vi "Flatten Cluster To CfgTable(with DataName).vi"(8 "error in (no error)":errorcluster, 10 "ParentName":string, 11 "Cluster Configuration Typedef":variant) -> (0 "error out":errorcluster, 2 "CfgTable Row Header":string[](array[string]), 3 "CfgTable Row":string[](array[string]))   [LabVIEW 2017, in "ClusterCfgTable.lvlib"]
uses:
  ClusterCfgTable.lvlib
panel:
  in  "ConfigStrings Typedef":string[](array[string])
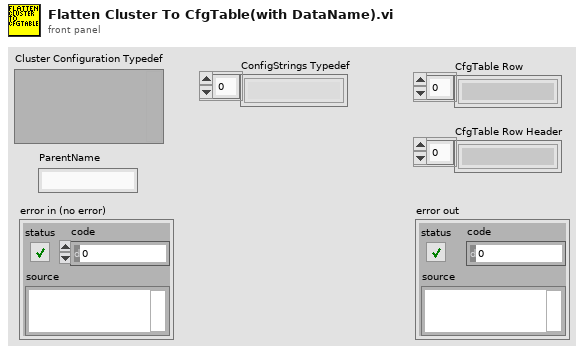
[diagram p1: front panel]
types:
  T1 = typedef "Type Descriptor Enumeration__ogtk.ctl" = enum8{"<Null>", "I8", "I16", "I32", "I64", "U8", "U16", "U32", "U64", "SGL", "DBL", "EXT", "CSG", "CDB", "CXT", "0x0F", "0x10", "0x11", "0x12", "0x13", "0x14", "Enum U8", "Enum U16", "Enum U32", "Enum U64", "SGL PQ", "DBL PQ", "EXT PQ", "CSG PQ", "CDB PQ", "CXT PQ", "0x1F", "0x20", "Boolean", "0x22", "0x23", "0x24", "0x25", "0x26", "0x27", "0x28", "0x29", "0x2A", "0x2B", "0x2C", "0x2D", "0x2E", "0x2F", "String", "0x31", "Path", "Pict", "0x34", "0x35", "0x36", "DAQ", "0x38", "0x39", "0x3A", "0x3B", "0x3C", "0x3D", "0x3E", "0x3F", "Array", "0x41", "0x42", "0x43", "0x44", "0x45", "0x46", "0x47", "0x48", "0x49", "0x4A", "0x4B", "0x4C", "0x4D", "0x4E", "0x4F", "Cluster", "0x51", "0x52", "Variant", "Waveform", "0x55", "0x56", "0x57", "0x58", "0x59", "0x5A", "0x5B", "0x5C", "0x5D", "0x5E", "0x5F", "0x60", "0x61", "0x62", "0x63", "0x64", "0x65", "0x66", "0x67", "0x68", "0x69", "0x6A", "0x6B", "0x6C", "0x6D", "0x6E", "0x6F", "Refnum"}
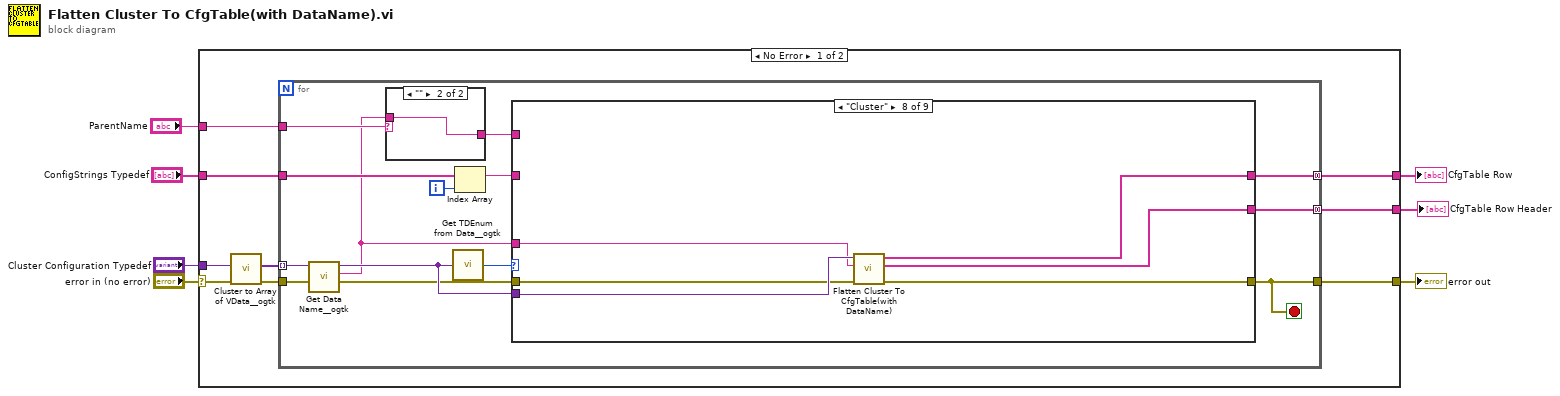
[diagram p0: block diagram]
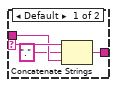
[diagram p2: hidden frame]
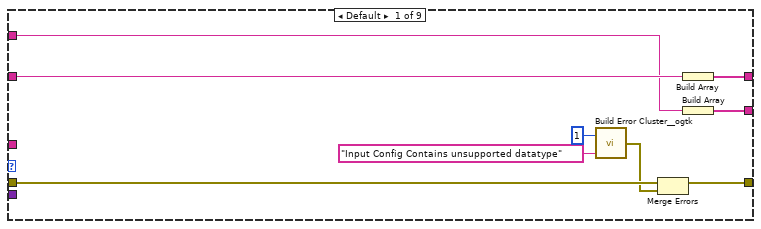
[diagram p3: hidden frame]
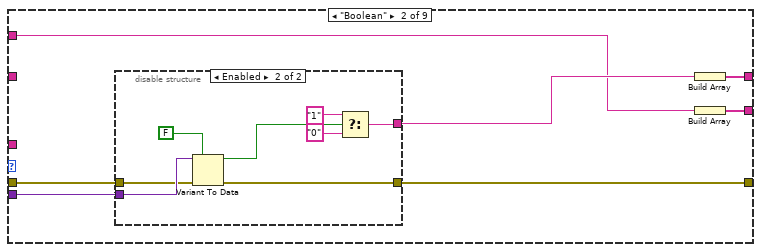
[diagram p4: hidden frame]
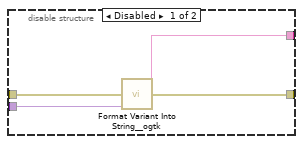
[diagram p5: hidden frame]
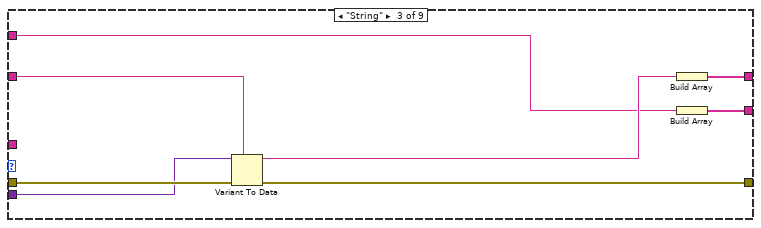
[diagram p6: hidden frame]
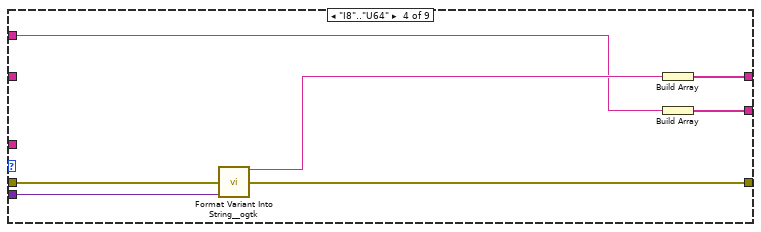
[diagram p7: hidden frame]
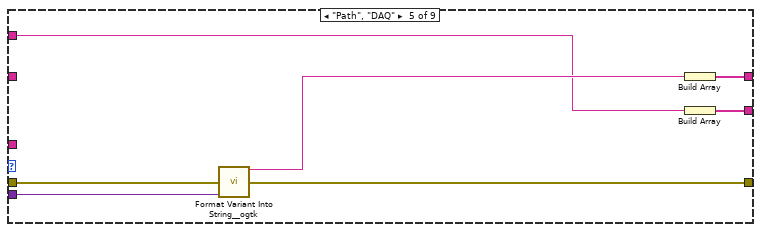
[diagram p8: hidden frame]
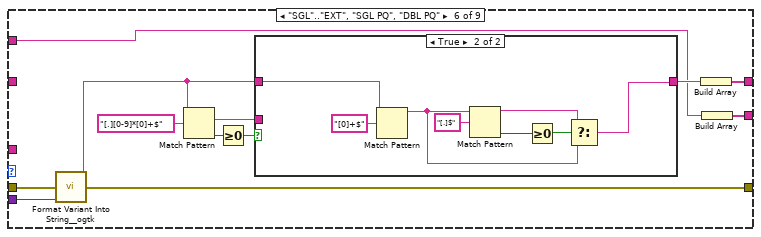
[diagram p9: hidden frame]
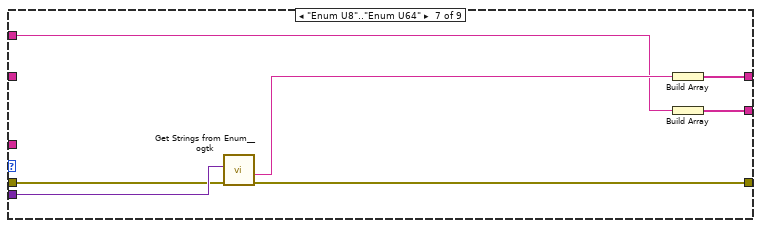
[diagram p11: hidden frame]
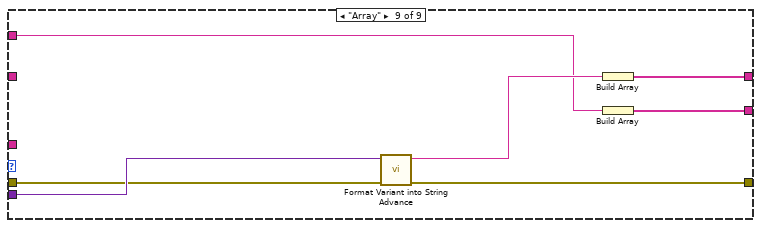
[diagram p12: hidden frame]
diagram:
  n1 = case shown="No Error" "error in (no error)" {
    selector: "error in (no error)" -> [w14 w128]
    tunnel: [w16 w128] -> w7
    tunnel: "Cluster Configuration Typedef" -> [w12 _]
    tunnel: [w11 w127] -> w4
    tunnel: "ConfigStrings Typedef" -> [w10 w127]
    tunnel: "ParentName" -> [w9 _]
    tunnel: [w8 _] -> w1
    frame No Error {
      n2 = call <userlib>:"Cluster to Array of VData__ogtk.vi"("error in (no error)"=w14, "Cluster"=w12) -> ("error out"=w15:errorcluster, "Array of VData"=w13:variant[])  [unwired: 8 in]
      n3 = for {
        tunnel: w13 -> [w29] mode=indexing
        tunnel: w15 -> [w22]
        tunnel: [w28] -> w16
        tunnel: [w27] -> w11 mode=concatenating
        tunnel: w10 -> [w26]
        tunnel: w9 -> [w20]
        tunnel: [w17] -> w8 mode=concatenating
        i -> [w24]
        stop <- w28 stop-if-true
        n4 = call <userlib>:"Get Data Name__ogtk.vi"("error in (no error)"=w22, "Data"=w29) -> ("error out"=w21:errorcluster, "Data Name"=w19:string, "Data dup"=w23:variant)  [unwired: 7 in]
        n5 = case shown="\"\"" w20 {
          selector: w20 -> [w34 _]
          tunnel: w19 -> [w33 w35]
          tunnel: [w31 w35] -> w18
          frame Default {
            n6 = Concatenate Strings(w34, "." ("string"), w33) -> (w31:string)
          }
          frame "" {
          }
        }
        n7 = call <userlib>:"Get TDEnum from Data__ogtk.vi"("Data"=w23) -> ("Type Descriptor Enumeration"=w30:T1)  [unwired: 4 in]
        n8 = Index Array(array=w26, index=w24) -> (element=w25:string)
        n9 = case shown="\"Cluster\"" w30 {
          tunnel: w23 -> [_ w50 w69 w76 w83 w91 w113 w119 w126]
          tunnel: w21 -> [w44 w51 w71 w78 w85 w92 w112 w117 w122]
          tunnel: [w43 w48 w70 w77 w84 w90 w110 w116 w123] -> w28
          tunnel: [w38 w47 w66 w74 w81 w88 w109 w118 w124] -> w27
          tunnel: w25 -> [w39 _ w68 _ _ _ _ _ _]
          tunnel: w19 -> [_ _ _ _ _ _ _ w115 _]
          tunnel: w18 -> [w37 w46 w65 w73 w80 w87 w108 _ w121]
          tunnel: [w36 w45 w64 w72 w79 w86 w107 w114 w120] -> w17
          frame Default {
            n10 = call <userlib>:"Build Error Cluster__ogtk.vi"("String to Prepend to source (\"\")"="Input Config Contains unsupported datatype" ("String to Prepend to source (\"\")"), "code"=1) -> ("error out"=w42:errorcluster)
            n11 = Merge Errors(w44, w42) -> (w43:errorcluster)
            n12 = Build Array(w39) -> (w38:string[])
            n13 = Build Array(w37) -> (w36:string[])
          }
          frame "Boolean" {
            n14 = disable-structure shown="Enabled" {
              disable-tunnel: w50 -> [w55 w63]
              disable-tunnel: w51 -> [w54 w62]
              disable-tunnel: [w53 w61] -> w48
              disable-tunnel: [w52 w58] -> w49
              frame Disabled {
                n15 = call <userlib>:"Format Variant Into String__ogtk.vi"("error in (no error)"=w54, "Variant"=w55) -> ("Output String"=w52:string, "error out"=w53:errorcluster)  [unwired: 12 in]
              }
              frame Enabled {
                n16 = Variant To Data(error in=w62, type=FALSE, Variant=w63) -> (data=w59:bool, error out=w61:errorcluster)
                n17 = Select(t="1", s=w59, f="0") -> (s? t:f=w58:string)
              }
            }
            n18 = Build Array(w49) -> (w47:string[])
            n19 = Build Array(w46) -> (w45:string[])
          }
          frame "String" {
            n20 = Variant To Data(error in=w71, type=w68, Variant=w69) -> (data=w67:string, error out=w70:errorcluster)
            n21 = Build Array(w67) -> (w66:string[])
            n22 = Build Array(w65) -> (w64:string[])
          }
          frame "I8".."U64" {
            n23 = call <userlib>:"Format Variant Into String__ogtk.vi"("error in (no error)"=w78, "Variant"=w76) -> ("Output String"=w75:string, "error out"=w77:errorcluster)  [unwired: 12 in]
            n24 = Build Array(w75) -> (w74:string[])
            n25 = Build Array(w73) -> (w72:string[])
          }
          frame "Path", "DAQ" {
            n26 = call <userlib>:"Format Variant Into String__ogtk.vi"("error in (no error)"=w85, "Variant"=w83) -> ("Output String"=w82:string, "error out"=w84:errorcluster)  [unwired: 12 in]
            n27 = Build Array(w82) -> (w81:string[])
            n28 = Build Array(w80) -> (w79:string[])
          }
          frame "SGL".."EXT", "SGL PQ", "DBL PQ" {
            n29 = call <userlib>:"Format Variant Into String__ogtk.vi"("error in (no error)"=w92, "Variant"=w91) -> ("Output String"=w94:string, "error out"=w90:errorcluster)  [unwired: 12 in]
            n30 = Match Pattern(string=w94, regular expression="[.][0-9]*[0]+$") -> (match substring=w93:string, offset past match=w96:i32)  [unwired: 1 in, 2 out]
            n31 = Greater Or Equal To 0?(x=w96) -> (x >= 0?=w95:bool)
            n32 = case shown="True" w95 {
              tunnel: [w98 w106] -> w89
              tunnel: w94 -> [w98 w104]
              tunnel: w93 -> [_ _]
              frame False {
              }
              frame True {
                n33 = Match Pattern(string=w104, regular expression="[0]+$") -> (before substring=w103:string)  [unwired: 1 in, 3 out]
                n34 = Match Pattern(string=w103, regular expression="[.]$") -> (before substring=w99:string, offset past match=w101:i32)  [unwired: 1 in, 2 out]
                n35 = Greater Or Equal To 0?(x=w101) -> (x >= 0?=w100:bool)
                n36 = Select(t=w99, s=w100, f=w103) -> (s? t:f=w106:string)
              }
            }
            n37 = Build Array(w89) -> (w88:string[])
            n38 = Build Array(w87) -> (w86:string[])
          }
          frame "Enum U8".."Enum U64" {
            n39 = call <userlib>:"Get Strings from Enum__ogtk.vi"("error in (no error)"=w112, "Enum"=w113) -> ("error out"=w110:errorcluster, "String Value"=w111:string)  [unwired: 6 in, 2 out]
            n40 = Build Array(w111) -> (w109:string[])
            n41 = Build Array(w108) -> (w107:string[])
          }
          frame "Cluster" {
            n42 = call "Flatten Cluster To CfgTable(with DataName).vi"("error in (no error)"=w117, "ParentName"=w115, "Cluster Configuration Typedef"=w119) -> ("error out"=w116:errorcluster, "CfgTable Row Header"=w114:string[], "CfgTable Row"=w118:string[])  [unwired: 6 in]
          }
          frame "Array" {
            n43 = call "Format Variant into String Advance.vi"("error in (no error)"=w122, "Variant"=w126) -> ("error out"=w123:errorcluster, "Data"=w125:string)  [unwired: 7 in, 1 out]
            n44 = Build Array(w125) -> (w124:string[])
            n45 = Build Array(w121) -> (w120:string[])
          }
        }
      }
    }
    frame Error {
    }
  }
  "CfgTable Row" <- w4
  "error out" <- w7
  "CfgTable Row Header" <- w1
